vi "Coerce to Zero.vi"(10 "Number IN":i32) -> (2 "Number OUT":i32)   [LabVIEW 2019]
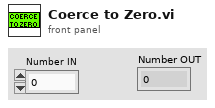
[diagram p1: front panel]
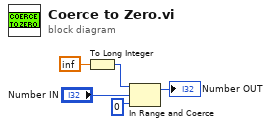
[diagram p0: block diagram]
diagram:
  n1 = To Long Integer(number=inf) -> (32bit integer=w3:i32)
  n2 = In Range and Coerce(upper limit=w3, x="Number IN", lower limit=0) -> (coerced(x)=→"Number OUT":i32)  [unwired: 1 out]
